vi "catch file error.vi"(8 "failure in":T3 {"code" format="%.0x"}) -> (0 "failure out":T3 {"code" format="%.0x"}, 1 "severity":T2, 2 "file error":T1, 3 "file failure?":bool, 5 "file failure":T3 {"code" format="%.0x"})   [LabVIEW 2013, in "file errors.lvlib"]
uses:
  file errors.lvlib
  failure.ctl
  severity.ctl
  file error.ctl
  failure.lvlib
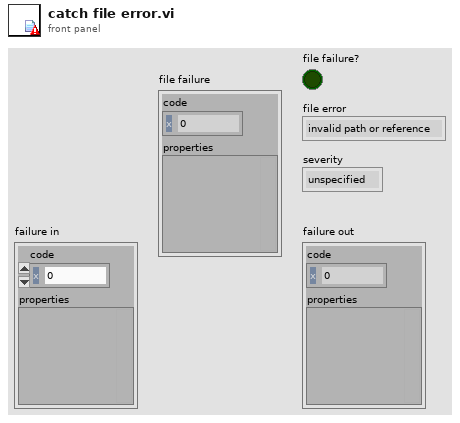
[diagram p1: front panel]
types:
  T1 = typedef "file errors.lvlib/file error.ctl" = enum16{"invalid path or reference", "end of file", "file already opened", "generic file error", "file not found", "permissions invalid", "disk full", "duplicate path", "too many open file handles", "useless generic error"}
  T2 = typedef "failure.lvlib/severity.ctl" = enum8{"unspecified", "informational", "operation failed", "data corruption", "system corruption", "critical unknown state"}
  T3 = typedef "failure.lvlib/failure.ctl" = cluster{"code":i32, "properties":variant}
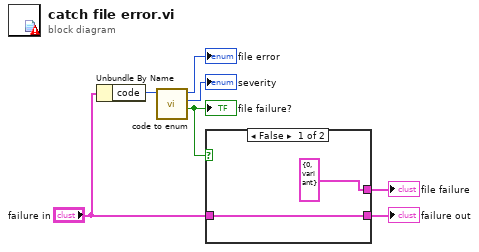
[diagram p0: block diagram]
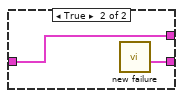
[diagram p2: hidden frame]
diagram:
  n1 = Unbundle By Name("failure in") -> ("code"=w7:i32)
  n2 = call "code to enum.vi"("code"=w7) -> ("valid?"=w6:bool, "severity"=→"severity":T2, "file error"=→"file error":T1)  [unwired: 8 in]
  "file failure?" <- w6
  n3 = case shown="False" w6 {
    tunnel: "failure in" -> [w9 w11]
    tunnel: [T3 {"code"=0, "properties"=variant} ("failure in") w11] -> w4
    tunnel: [w9 w10] -> w1
    frame False {
    }
    frame True {
      n4 = call "new failure.vi"() -> ("failure"=w10:T3)  [unwired: 11 in]
    }
  }
  "failure out" <- w1
  "file failure" <- w4
